vi "Read Parameters.vi"(8 "error in (no error)":errorcluster, 11 "Mag Lab Parameters in":refnum<class "Mag Lab Parameters.lvclass">) -> (0 "error out":errorcluster, 2 "Parameters":variant, 3 "Mag Lab Parameters out":refnum<class "Mag Lab Parameters.lvclass">)   [LabVIEW 2015, in "Mag Lab Parameters.lvclass"]
uses:
  Mag Lab Parameters.lvclass
  Mag Lab Parameters.lvclass/Mag Lab Parameters.ctl
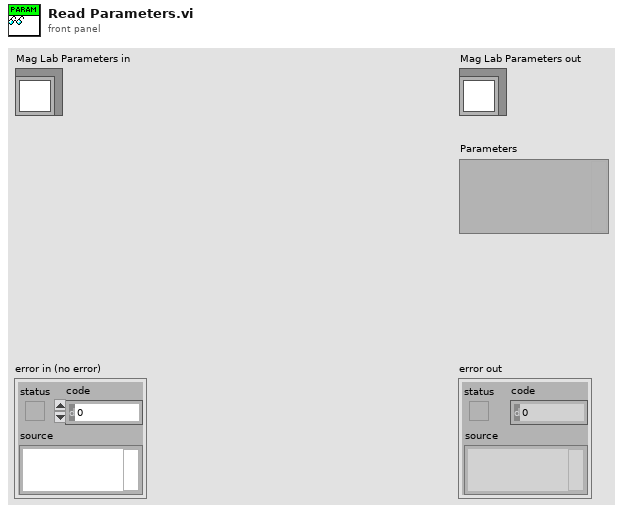
[diagram p1: front panel]
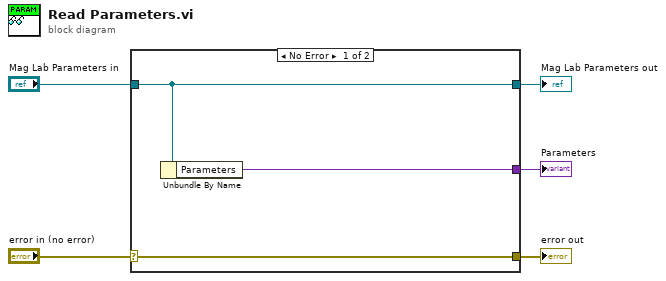
[diagram p0: block diagram]
diagram:
  n1 = case shown="No Error" "error in (no error)" {
    selector: "error in (no error)" -> [w8 w9]
    tunnel: [w8 w9] -> w4
    tunnel: [w7 w10] -> w2
    tunnel: "Mag Lab Parameters in" -> [w7 w10]
    tunnel: [w6 _] -> w1
    frame No Error {
      n2 = Unbundle By Name(w7) -> ("Parameters"=w6:variant)
    }
    frame Error {
    }
  }
  "error out" <- w4
  "Mag Lab Parameters out" <- w2
  "Parameters" <- w1
